vi "Write name.vi"(8 "error in (no error)":errorcluster, 10 "guiderName":string, 11 "GuiderName.lvclass in":refnum<class "GuiderName.lvclass">) -> (0 "error out":errorcluster, 3 "GuiderName.lvclass out":refnum<class "GuiderName.lvclass">)   [LabVIEW 2014, in "TCSDataDefinitions.lvlib" / "TCSGuiderCommand.lvlib" / "GuiderName.lvclass"]
uses:
  GuiderName.lvclass
  GuiderName.lvclass/GuiderName.ctl
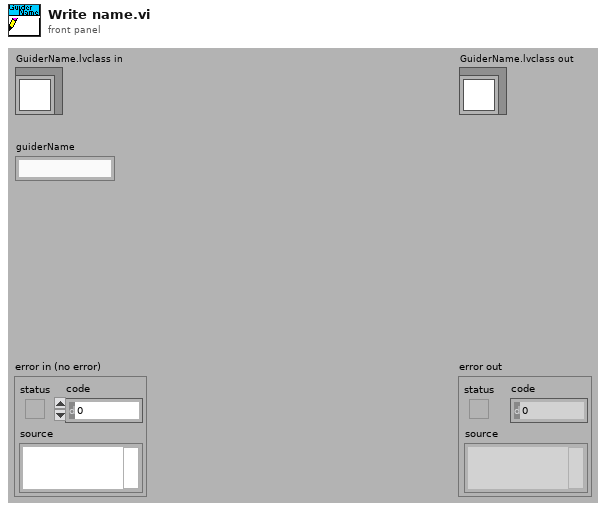
[diagram p1: front panel]
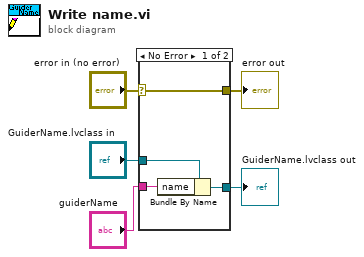
[diagram p0: block diagram]
diagram:
  n1 = case shown="No Error" "error in (no error)" {
    selector: "error in (no error)" -> [w9 w10]
    tunnel: [w9 w10] -> w4
    tunnel: [w7 w11] -> w2
    tunnel: "GuiderName.lvclass in" -> [w8 w11]
    tunnel: "guiderName" -> [w6 _]
    frame No Error {
      n2 = Bundle By Name(cluster=w8, "name"=w6) -> (w7:refnum<class "GuiderName.lvclass">)
    }
    frame Error {
    }
  }
  "error out" <- w4
  "GuiderName.lvclass out" <- w2
